vi "tcs shm put Sample kernel Track Ref Sys LV.vi"(8 "error in (no error)":errorcluster, 11 "kernel_TrackRefSys_Ctl":T1) -> (0 "error out":errorcluster, 2 "function return":i32, 3 "kernel_TrackRefSys_Ctl out":T1)   [LabVIEW 2016, in "SALLV_tcs.lvlib"]
doc: "int tcs_shm_putSample_kernel_TrackRefSysLV(tcs_kernel_TrackRefSysLV *kernel_TrackRefSys_Ctl );"
uses:
  SALLV_tcs.lvlib
  SALLV_tcs.so
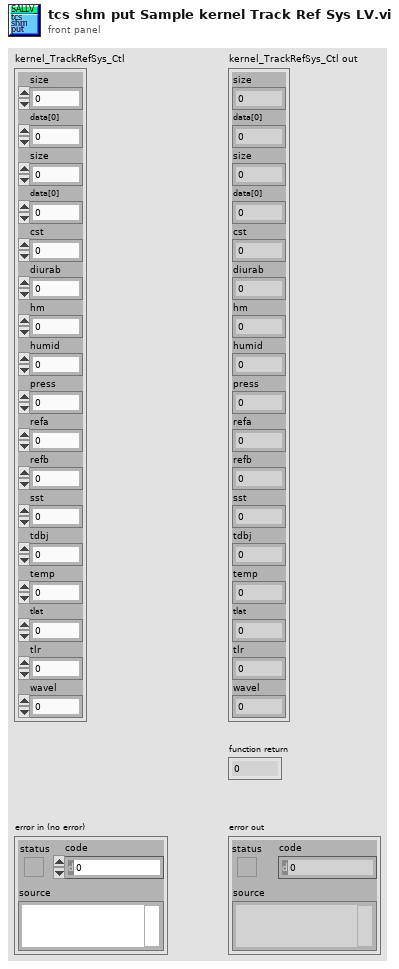
[diagram p1: front panel]
types:
  T1 = cluster{"size":i32, "data[0]":sgl, "size":i32, "data[0]":sgl, "cst":sgl, "diurab":sgl, "hm":sgl, "humid":sgl, "press":sgl, "refa":sgl, "refb":sgl, "sst":sgl, "tdbj":sgl, "temp":sgl, "tlat":sgl, "tlr":sgl, "wavel":sgl}
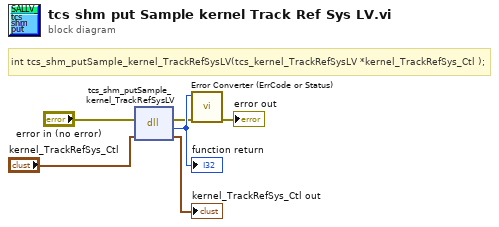
[diagram p0: block diagram]
diagram:
  # "int tcs_shm_putSample_kernel_TrackRefSysLV(tcs_kernel_TrackRefSysLV *kernel_TrackRefSys_Ctl );"
  n1 = dll-call lib="home/andres/Desktop/SALLV_tcs/SALLV_tcs.*" fn="tcs_shm_putSample_kernel_TrackRefSysLV"(error in="error in (no error)", "kernel_TrackRefSys_Ctl"="kernel_TrackRefSys_Ctl") -> (error out=w2:errorcluster, w6:i32, "kernel_TrackRefSys_Ctl"=→"kernel_TrackRefSys_Ctl out":T1)  [unwired: 2 in, 1 out]
  "function return" <- w6
  n2 = call "Error Converter (ErrCode or Status).vi"("error in (no error)"=w2, "error code"=w6) -> ("error out"=→"error out":errorcluster)  [unwired: 9 in]
